vi "3-1.vi"() -> ()   [LabVIEW 2019, in "AoC2022.lvlib"]
uses:
  AoC2022.lvlib
panel:
  out "sum":u32
  out "string 2":string
  out "string":string
  out "Array":u8[](array[numeric])
  out "subarray 2":u8[](array[numeric])
  out "subarray":u8[](array[numeric])
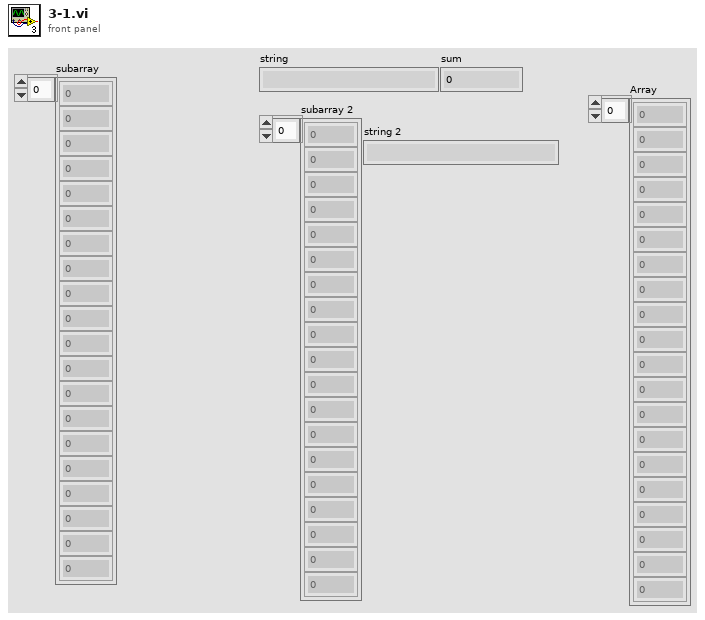
[diagram p1: front panel]
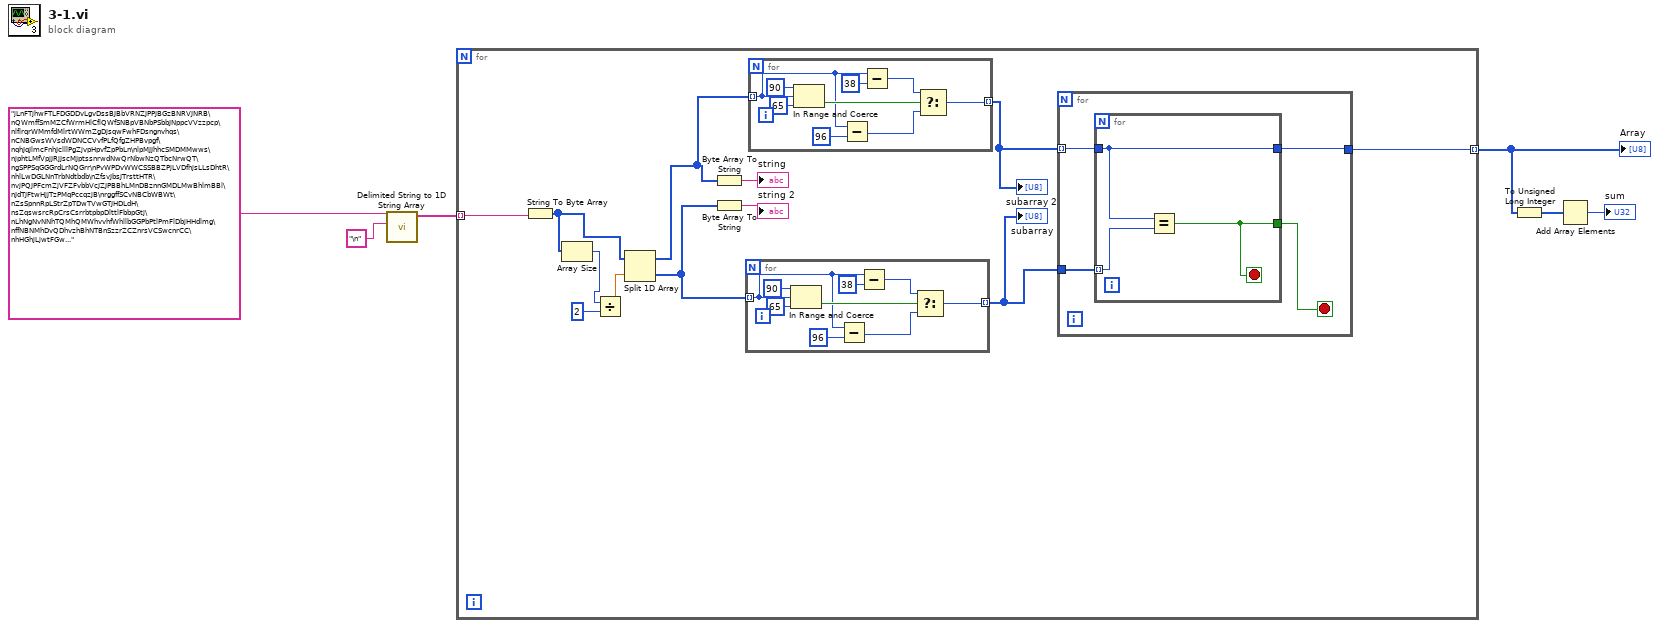
[diagram p0: block diagram]
diagram:
  n1 = call <vilib>:"Delimited String to 1D String Array.vi"("delimiter"="\n", "delimited string"="jLnFTjhwFTLFDGDDvLgvDssBJBbVRNZJPPJBGzBNRVJNRB\nQWmffSmMZCfWrmHlCflQWfSNBpVBNbPSbbJNppcVVzzpcp\nlflrqrWMmfdMlrtWWmZgDjsqwFwhFDsngnvhqs\nCNBGwsWVsdWDNCCVvfPLfQfgZHPBvpgf\nqhJqJlmcFnhJclllPgZjvpHpvfZpPbLn\nlpMJJhhcSMDMMwws\njphtLMfVpjJRjJscMJptssnrwdNwQrNbwNzQTbcNrwQT\ngSPPSqGGGrdLrNQGrr\nPvWPDvWWCSSBBZPjLVDfhjsLLsDhtR\nhlLwDGLNnTrbNdtbdb\nZfsvJbsJTrsttHTR\nvjPQJPFcmZjVFZFvbbVcJZJPBBhLMnDBznnGMDLMwBhlmBBl\nJdTJFtwHjJTzPMqPccqzjB\nrggffSCvNBCbWBWt\nZsSpnnRpLStrZpTDwTVwGTJHDLdH\nsZqswsrcRpCrsCsrrbtpbpDlttlFbbpGtj\nLhNgNvNNhTQMhQMWhvvhfWhllbGGPbPtlPmFlDbjHHdlmg\nffNBNMhDvQDhvzhBhNTBnSzzrZCZnrsVCSwcnrCC\nhHGhjLjwtFGw...") -> ("string array"=w4:string[])  [unwired: 9 in]
  n2 = for {
    tunnel: w4 -> [w18] mode=indexing
    tunnel: [w17] -> w3 mode=indexing
    n3 = String To Byte Array(string=w18) -> (unsigned byte array=w9:u8[])
    n4 = Array Size(array=w9) -> (size(s)=w12:i32)
    n5 = Divide(x=w12, y=2) -> (x/y=w10:dbl)
    n6 = Split 1D Array(array=w9, index=w10) -> (first subarray=w8:u8[], second subarray=w7:u8[])
    n7 = Byte Array To String(unsigned byte array=w8) -> (string=→"string":string)
    n8 = Byte Array To String(unsigned byte array=w7) -> (string=→"string 2":string)
    n9 = for {
      tunnel: w7 -> [w26] mode=indexing
      tunnel: [w29] -> w15 mode=indexing
      n10 = In Range and Coerce(upper limit=u8 90, x=w26, lower limit=u8 65) -> (In Range?=w32:bool)  [unwired: 1 out]
      n11 = Subtract(x=w26, y=u8 96) -> (x-y=w27:u8)
      n12 = Subtract(x=w26, y=u8 38) -> (x-y=w30:u8)
      n13 = Select(t=w30, s=w32, f=w27) -> (s? t:f=w29:u8)
    }
    "subarray" <- w15
    n14 = for {
      tunnel: w8 -> [w35] mode=indexing
      tunnel: [w38] -> w16 mode=indexing
      n15 = In Range and Coerce(upper limit=u8 90, x=w35, lower limit=u8 65) -> (In Range?=w41:bool)  [unwired: 1 out]
      n16 = Subtract(x=w35, y=u8 96) -> (x-y=w36:u8)
      n17 = Subtract(x=w35, y=u8 38) -> (x-y=w39:u8)
      n18 = Select(t=w39, s=w41, f=w36) -> (s? t:f=w38:u8)
    }
    "subarray 2" <- w16
    n19 = for {
      tunnel: w16 -> [w21] mode=indexing
      tunnel: w15 -> [w22]
      tunnel: [w19] -> w17
      stop <- w20 stop-if-true
      n20 = for {
        tunnel: w22 -> [w25] mode=indexing
        tunnel: w21 -> [w23]
        tunnel: [w24] -> w20
        tunnel: [w23] -> w19
        stop <- w24 stop-if-true
        n21 = Equal?(x=w23, y=w25) -> (x = y?=w24:bool)
      }
    }
  }
  "Array" <- w3
  n22 = To Unsigned Long Integer(number=w3) -> (unsigned 32bit integer=w2:u32[])
  n23 = Add Array Elements(numeric array=w2) -> (sum=→"sum":u32)
